vi "Configure Trigger (Communication - CMI).vi"(0 "VISA resource name":refnum<visa-resource-name>, 1 "Standard (20:DS4NA)":u16(ring)=20 items=["DS4NA"=20, "E4"=24, "STS3"=26, "STM1E"=27, "STM0_CMI"=60, "Custom"=70], 2 "Bit Rate (1.544Mb/s)":dbl=1544000.0, 3 "Pulse Form (0:1)":u16(ring) items=["+1", "0", "-1", "Eye"], 5 "Source (0:Channel1)":u16(ring) items=["Channel1", "Channel2", "Channel3", "Channel4"], 7 "Trigger Level (0V)":dbl, 9 "Source Type (0:Data)":u16(ring) items=["Data", "Clock"], 11 "error in (no error)":errorcluster, 12 "Clock Polarity (0:Positive)":u16(ring) items=["Positive", "Negative"]) -> (4 "VISA resource name out":refnum<visa-resource-name>, 15 "error out":errorcluster)   [LabVIEW 2011, in "Tektronix 7000 Series.lvlib"]
doc: "Configures Communication trigger settings for an oscilloscope.A trigger occurs when a communications signal is found. Supports CMI encoded communications signals.\n\nTDS5000,TDS5000B series oscilloscopes don't support this trigger."
uses:
  Tektronix 7000 Series.lvlib
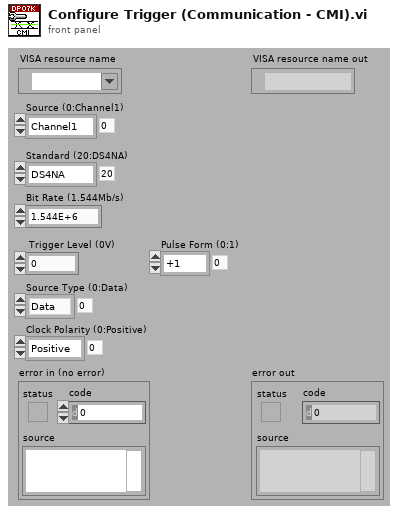
[diagram p1: front panel]
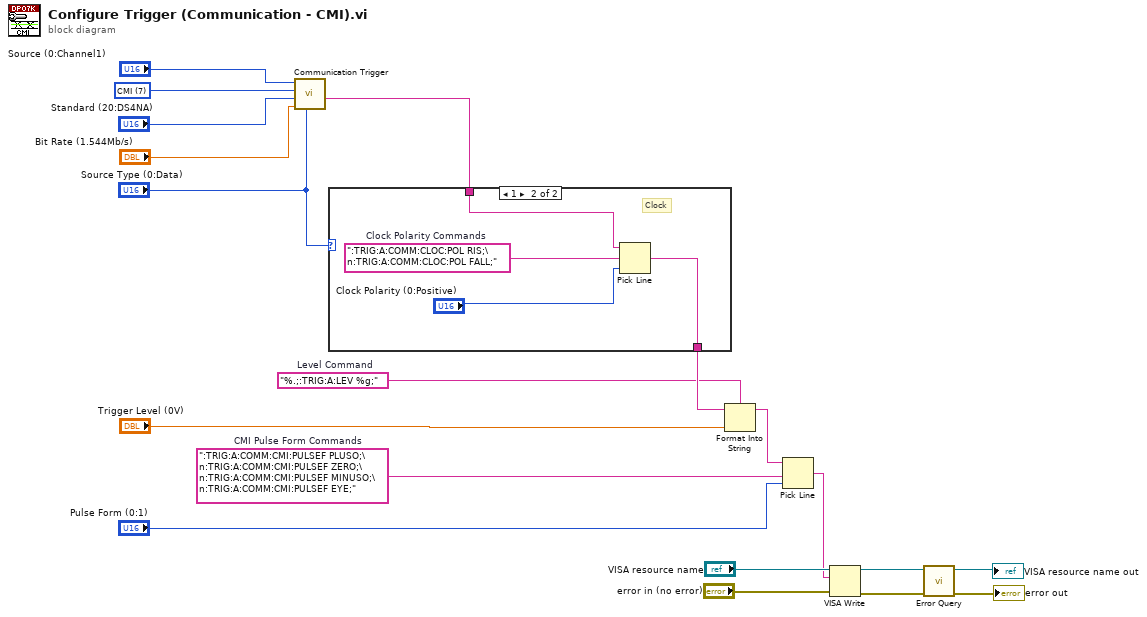
[diagram p0: block diagram]
diagram:
  w9 = ":TRIG:A:COMM:CMI:PULSEF PLUSO;\n:TRIG:A:COMM:CMI:PULSEF ZERO;\n:TRIG:A:COMM:CMI:PULSEF MINUSO;\n:TRIG:A:COMM:CMI:PULSEF EYE;"  # CMI Pulse Form Commands
  w12 = "%.;:TRIG:A:LEV %g;"  # Level Command
  w16 = u16 7 items=["NRZ", "MLT3", "AMI", "HDB3", "B3ZS", "B6ZS", "B8ZS", "CMI"] ("Coding (0:NRZ)")
  n1 = call "Communication Trigger.vi"("Source Type (0:Data)"="Source Type (0:Data)", "Bit Rate (1.544E6Mb/s)"="Bit Rate (1.544Mb/s)", "Standard (0:ATAG1)"="Standard (20:DS4NA)", "Coding (0:NRZ)"=w16, "Source (0:Channel1)"="Source (0:Channel1)") -> ("Output String"=w18:string)  [unwired: 6 in]
  n2 = case shown="1" "Source Type (0:Data)" {
    tunnel: w18 -> [w20 w24]
    tunnel: [w20 w23] -> w19
    frame 0, Default {
      # "Data"
    }
    frame 1 {
      w22 = ":TRIG:A:COMM:CLOC:POL RIS;\n:TRIG:A:COMM:CLOC:POL FALL;"  # Clock Polarity Commands
      # "Clock"
      n3 = Pick Line(string ("")=w24, multi-line string=w22, line index="Clock Polarity (0:Positive)") -> (output string=w23:string)
    }
  }
  n4 = Format Into String(format string=w12, initial string=w19, "Trigger Level (0V)") -> (resulting string=w10:string)  [unwired: 1 in, 1 out]
  n5 = Pick Line(string ("")=w10, multi-line string=w9, line index="Pulse Form (0:1)") -> (output string=w1:string)
  n6 = VISA Write(VISA resource name="VISA resource name", write buffer=w1, error in (no error)="error in (no error)") -> (VISA resource name out=w6:refnum<visa-resource-name>, error out=w7:errorcluster)  [unwired: 1 out]
  n7 = call "Error Query.vi"("error in (no error)"=w7, "VISA resource name"=w6) -> ("error out"=→"error out":errorcluster, "VISA resource name out"=→"VISA resource name out":refnum<visa-resource-name>)  [unwired: 6 in, 2 out]
